vi "Red Pitaya Lockin Sweep.vi"(8 "Error In":errorcluster, 10 "Server port":u16=1002, 11 "Server address":string="192.168.1.100") -> (0 "Error Out":errorcluster)   [LabVIEW 2015]
uses:
  Mode.ctl
  Red Pitaya Parameters.ctl
  RP Command.ctl
panel:
  out "milliseconds to wait":u32=10
  in  "Desimate result":i32
  out "XY Graph":cluster{"Steps":dbl[], "Y":dbl[]}[](graph)
  out "FIFO counter":u32
  in  "Read FIFO":bool
  out "Waveform Chart 3":i32[](graph)
  out "Waveform Chart 2":i32[](graph)
  out "Waveform Chart":i32[](graph)
  out "last update, ms":i32
  in  "Controls":enum32{"Basic", "Advanced"}(tab)
  in  "Sweep":bool
  in  "Frequency step":dbl=100.0 format="%#_6p"
  in  "Stop frequency":dbl=802000.0 format="%#_6p"
  in  "Start frequency":dbl=800000.0 format="%#_6p"
  in  "Parameters":T1={"Ranges"=[20.0, 20.0], "Output frequency 1"=50000.0, "Output frequency 2"=50000.0, "Pre-trigger samples"=-100000, "Post-trigger samples"=67108864, "Desimation rate"=32, "Delayed start"=571428} {"Delayed start" format="0x%x (%d)"; "Post-trigger samples" format="0x%x (%d)"; "Pre-trigger samples" format="0x%x (%d)"; "Output frequency 2" format="%#_6p"; "Output frequency 1" format="%#_6p"; "Ranges" format="%#_12p"}
  out "CPU Temperature":dbl(slide)=48.847186279148 scale=0.0..100.0
  out "Temperature Chart":dbl(graph)=48.847186279148
  in  "Signal bits":i32=14
  in  "Read Temperature":bool=TRUE
  in  "Read trigger":bool
  in  "Start server":bool
  out "Server  output":string
  out "bytes written":i32=8
  out "Phase increment 1":u64=1717987
  out "Trigger state":bool
  in  "Mode":T2=enum."Digitizer"
  in  "Stop Server":bool
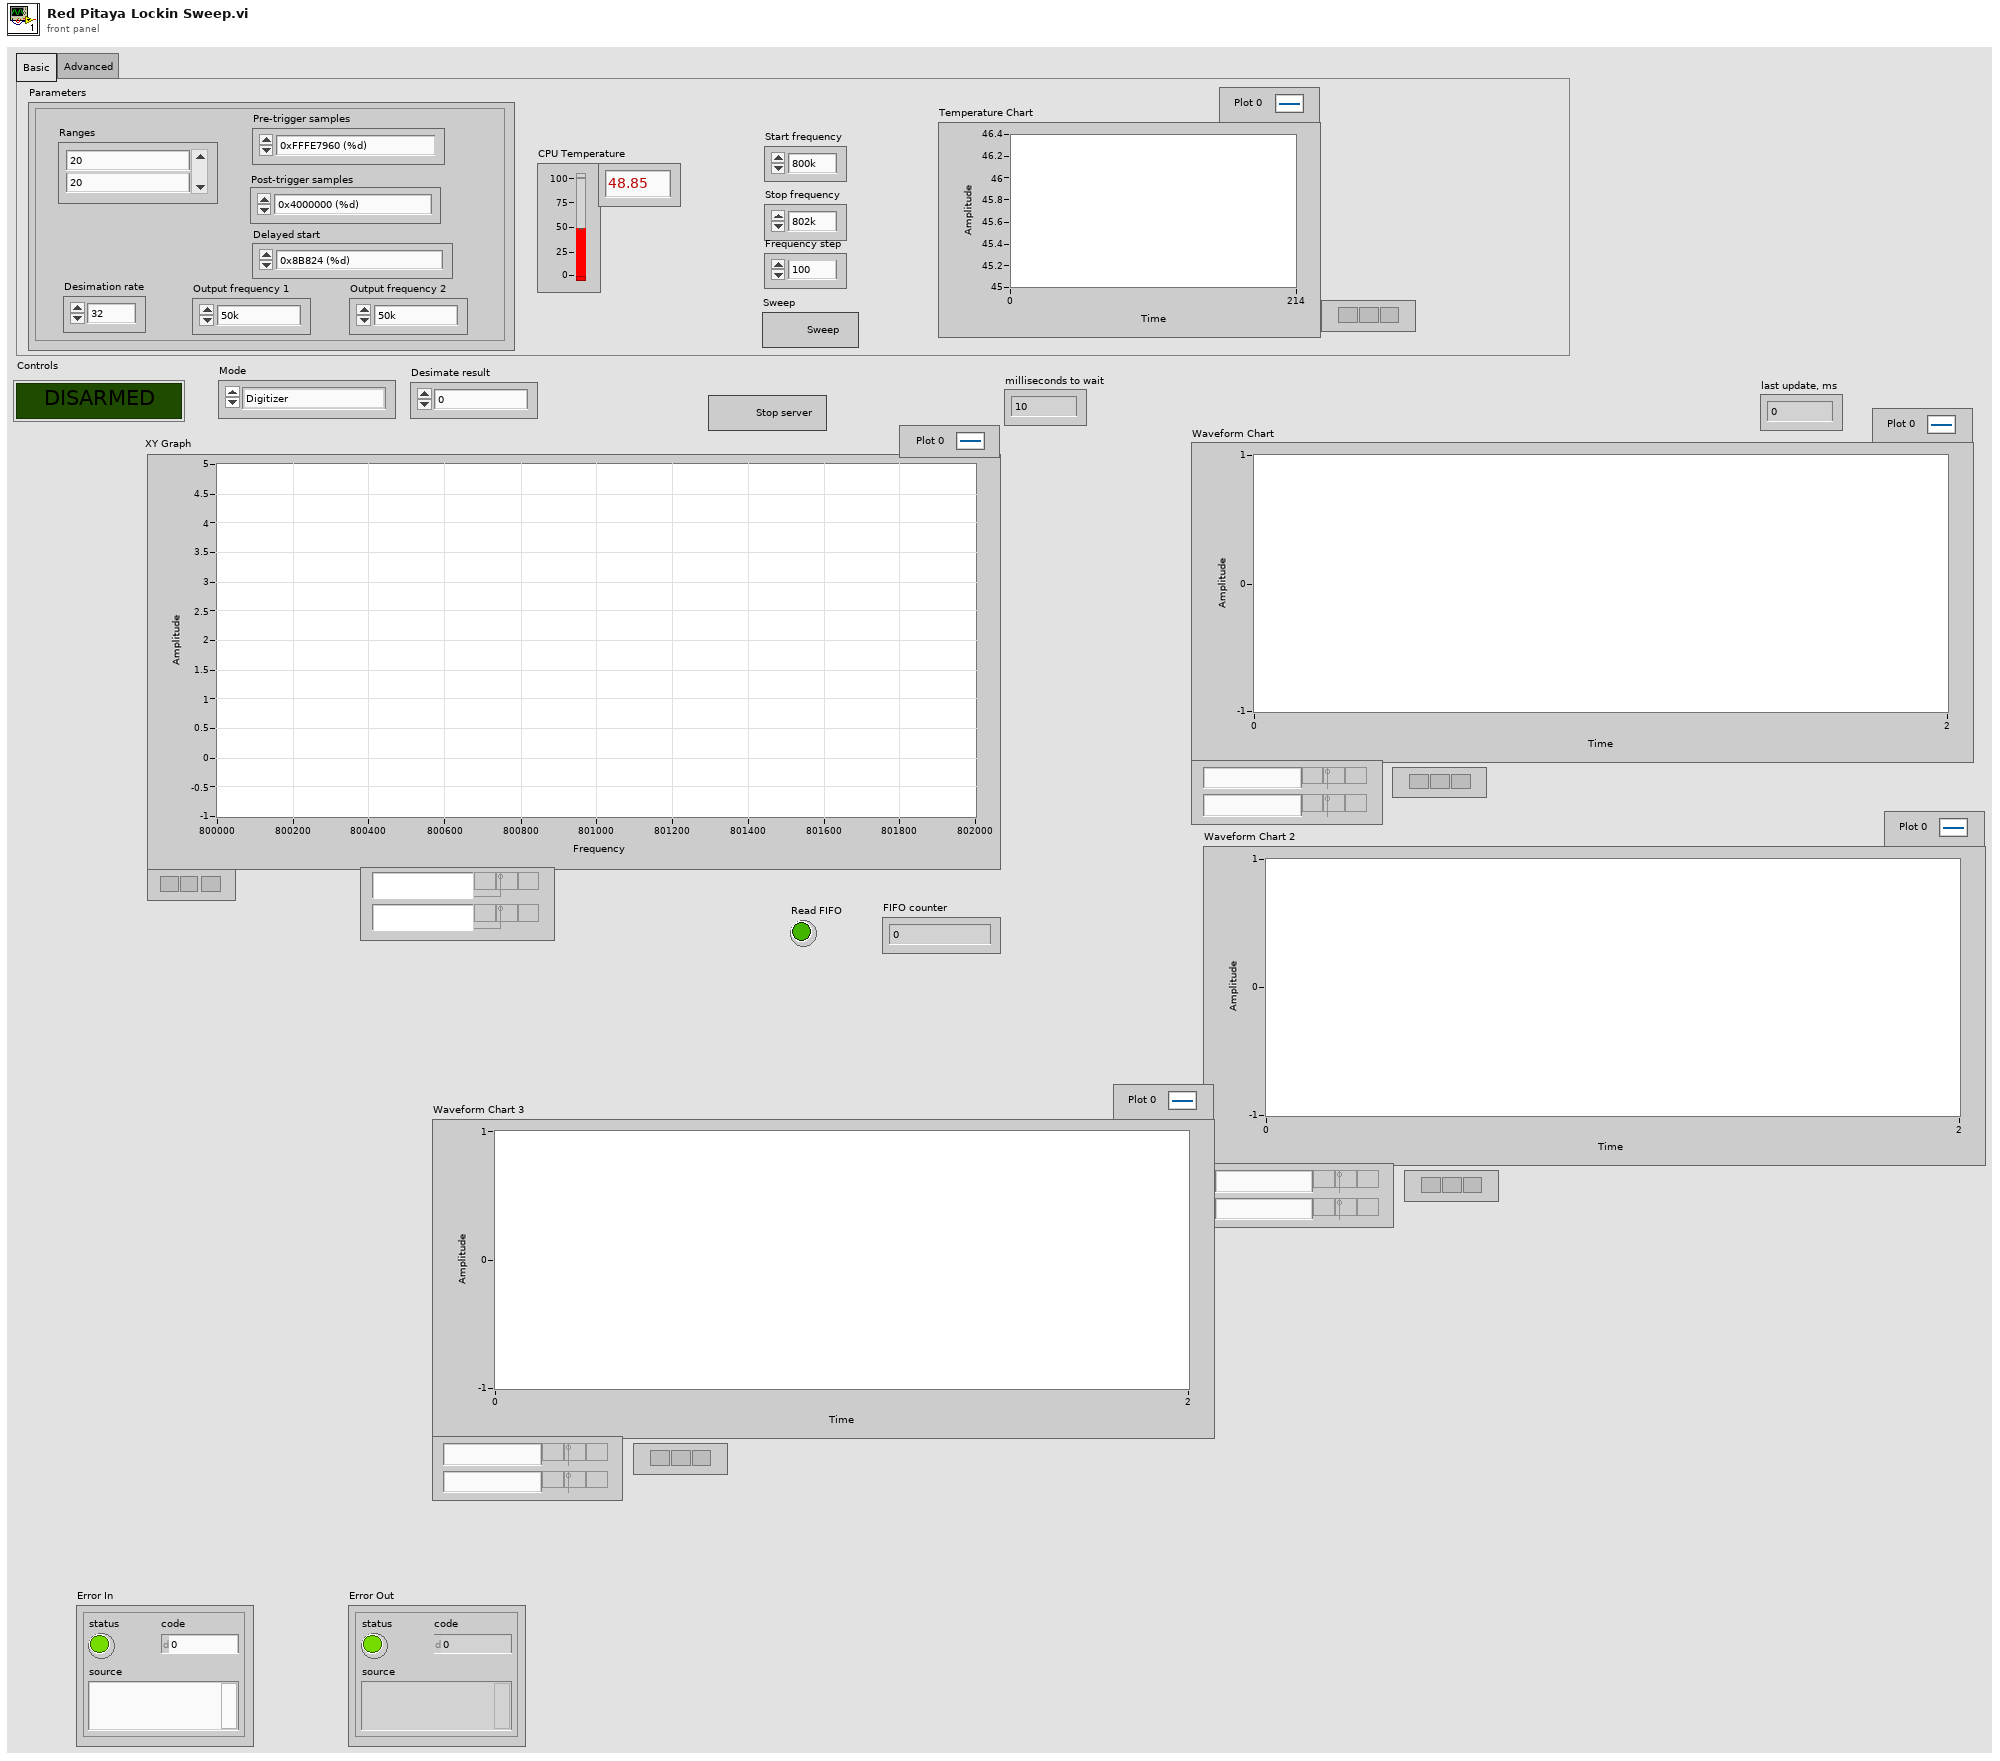
[diagram p1: front panel]
types:
  T1 = typedef "Red Pitaya Parameters.ctl" = cluster{"Ranges":dbl[], "Output frequency 1":dbl, "Output frequency 2":dbl, "Pre-trigger samples":i32, "Post-trigger samples":u64, "Desimation rate":u64, "Delayed start":u64}
  T2 = typedef "Mode.ctl" = enum16{"Filter", "Lockin test", "Snapshot test", "Digitizer", "Current-Voltage"}
  T3 = typedef "RP Command.ctl" = enum16{"Set frequency", "Arm and get data", "Stop server", "Get status", "Get temperature", "Set decimation", "Arm", "Software trigger", "Get whole buffer", "Get chunk", "System call", "Get config", "Set config", "Read FIFO", "Play pattern", "Set frequency batch"}
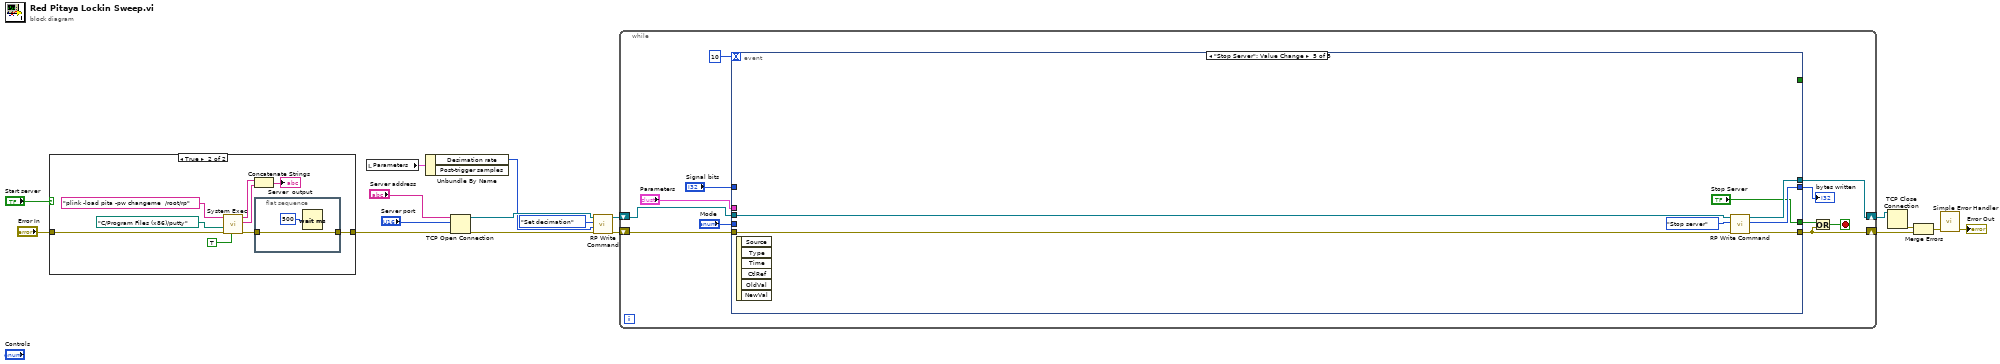
[diagram p0: block diagram]
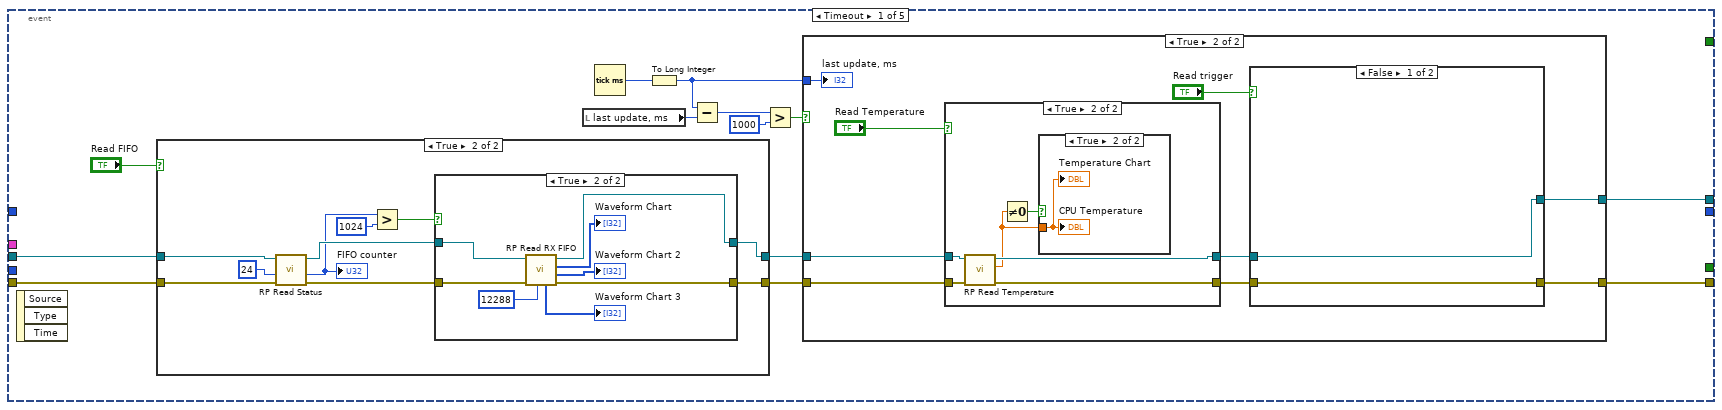
[diagram p3: hidden frame]
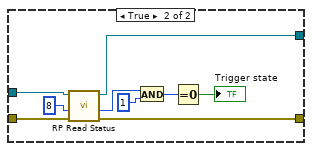
[diagram p7: hidden frame]
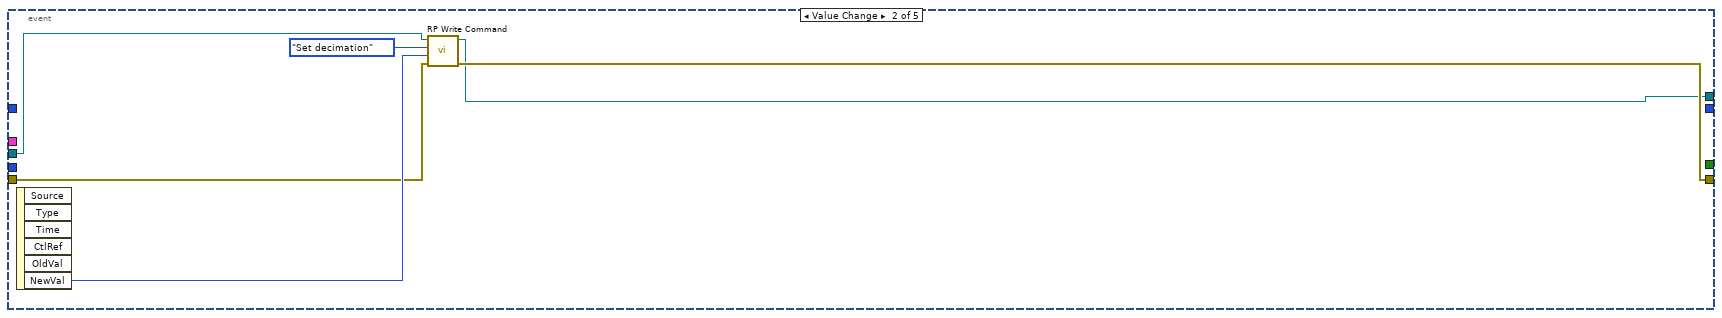
[diagram p10: hidden frame]
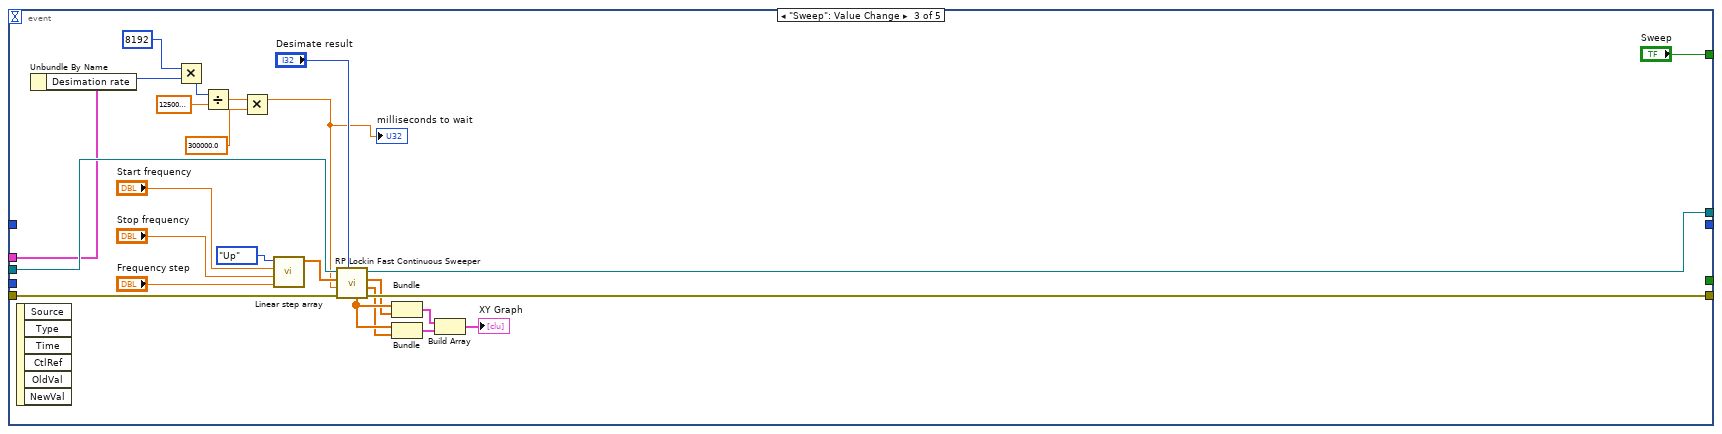
[diagram p11: hidden frame]
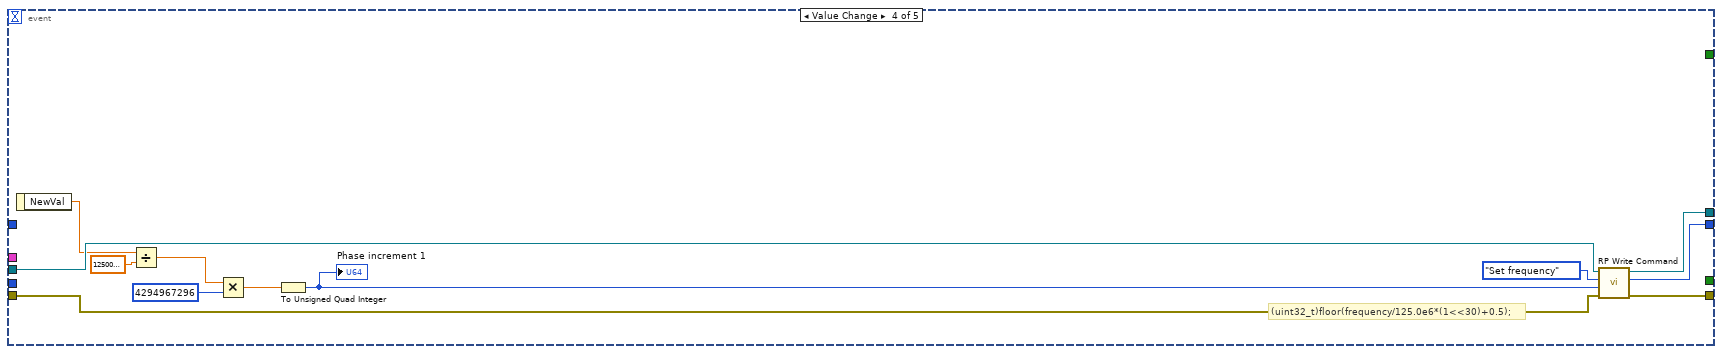
[diagram p12: hidden frame]
diagram:
  n1 = case shown="True" "Start server" {
    tunnel: [w18 w19] -> w9
    tunnel: "Error In" -> [w18 w21]
    frame False {
    }
    frame True {
      n2 = call <vilib>:"System Exec.vi"("run minimized? (F)"=TRUE, "error in (no error)"=w21, "working directory"=path "C:/Program Files (x86)/putty", "command line"="plink -load pita -pw changeme  /root/rp") -> ("error out"=w20:errorcluster, "standard error"=w23:string, "standard output"=w27:string)  [unwired: 4 in, 1 out]
      n3 = Concatenate Strings(w27, w23) -> (→"Server  output":string)
      n4 = flat-sequence {
        tunnel: w20 -> [w29]
        tunnel: [w29] -> w19
        frame #0 {
          n5 = Wait (ms)(milliseconds to wait=u32 500) -> ()  [unwired: 1 out]
        }
      }
    }
  }
  n6 = local read "Parameters"() -> (w6:T1)
  n7 = Unbundle By Name(w6) -> ("Desimation rate"=w3:u64)  [unwired: 1 out]
  n8 = TCP Open Connection(address="Server address", remote port or service name="Server port", error in (no error)=w9) -> (connection ID=w5:refnum<k5>, error out=w2:errorcluster)  [unwired: 2 in]
  n9 = call "RP Write Command.vi"("Error In"=w2, "Command payload"=w3, "Command number"=RP_Command."Set decimation", "connection ID"=w5) -> ("Error Out"=w1:errorcluster, "connection ID out"=w4:refnum<k5>)  [unwired: 5 in, 1 out]
  n10 = while {
    shift-right: [w38] -> w13
    shift-left: w4 -> [w39]
    shift-right: [w36] -> w12
    shift-left: w1 -> [w40]
    stop <- w34 stop-if-true
    n11 = event shown="[4] \"Stop Server\": Value Change" {
      selector: _ -> [_ _ _ _ _]
      dyn-events: _ -> [_ _ _ _ _]
      timeout: 10 -> [_ _ _ _ _]
      tunnel: w40 -> [w43 w110 w129 w145 w156]
      tunnel: w39 -> [w45 w109 w132 w144 w154]
      tunnel: [w53 w108 w130 w140 w153] -> w36
      tunnel: [w52 w107 w131 w141 w152] -> w38
      tunnel: [_ _ _ _ "Stop Server"] -> w35
      tunnel: [_ _ _ w139 w151] -> w37
      tunnel: "Mode" -> [_ _ _ _ _]
      tunnel: "Parameters" -> [_ _ w120 _ _]
      tunnel: "Signal bits" -> [_ _ _ _ _]
      tunnel: [_ _ "Sweep" _ _] -> _
      event Timeout {
        n12 = event-data() -> ()  [unwired: 1 in, 3 out]
        n13 = case shown="True" "Read FIFO" {
          tunnel: w45 -> [w54 w60]
          tunnel: [w54 w65] -> w44
          tunnel: w43 -> [w55 w63]
          tunnel: [w55 w64] -> w42
          frame False {
          }
          frame True {
            n14 = call "RP Read Status.vi"("Error In"=w63, "Status offset"=u64 24, "connection ID"=w60) -> ("Error Out"=w62:errorcluster, "Status response"=w58:u32, "connection ID out"=w61:refnum<k5>)  [unwired: 6 in]
            "FIFO counter" <- w58
            n15 = Greater?(x=w58, y=u32 1024) -> (0:w56:bool)
            n16 = case shown="True" w56 {
              tunnel: w61 -> [w66 w75]
              tunnel: [w66 w74] -> w65
              tunnel: [w67 w73] -> w64
              tunnel: w62 -> [w67 w69]
              frame False {
              }
              frame True {
                n17 = call "RP Read RX FIFO.vi"("FIFO Bytes per read"=12288, "Error In"=w69, "connection ID"=w75) -> ("Error Out"=w73:errorcluster, "Y"=→"Waveform Chart 2":i32[], "X"=→"Waveform Chart":i32[], "connection ID out"=w74:refnum<k5>, "F"=→"Waveform Chart 3":i32[])  [unwired: 4 in]
              }
            }
          }
        }
        n18 = local read "last update, ms"() -> (w50:i32)
        n19 = Tick Count (ms)() -> (millisecond timer value=w51:u32)
        n20 = To Long Integer(number=w51) -> (32bit integer=w46:i32)
        n21 = Subtract(x=w46, y=w50) -> (x-y=w49:i32)
        n22 = Greater?(x=w49, y=1000) -> (0:w47:bool)
        n23 = case shown="True" w47 {
          tunnel: w44 -> [w76 w85]
          tunnel: w42 -> [w77 w84]
          tunnel: [w77 w80] -> w53
          tunnel: [w76 w79] -> w52
          tunnel: w46 -> [_ w78]
          frame False {
          }
          frame True {
            n24 = case shown="True" "Read Temperature" {
              tunnel: w85 -> [w99 w104]
              tunnel: w84 -> [w98 w100]
              tunnel: [w99 w103] -> w82
              tunnel: [w98 w101] -> w81
              frame False {
              }
              frame True {
                n25 = call "RP Read Temperature.vi"("Error In"=w100, "connection ID"=w104) -> ("error out"=w101:errorcluster, "Thermometer"=w102:dbl, "connection ID out"=w103:refnum<k5>)  [unwired: 7 in]
                n26 = Not Equal To 0?(x=w102) -> (x != 0?=w105:bool)
                n27 = case shown="True" w105 {
                  tunnel: w102 -> [_ w106]
                  frame False {
                  }
                  frame True {
                    "CPU Temperature" <- w106
                    "Temperature Chart" <- w106
                  }
                }
              }
            }
            n28 = case shown="False" "Read trigger" {
              tunnel: w82 -> [w87 w96]
              tunnel: w81 -> [w88 w97]
              tunnel: [w88 w92] -> w80
              tunnel: [w87 w89] -> w79
              frame False {
              }
              frame True {
                n29 = call "RP Read Status.vi"("Error In"=w97, "Status offset"=u64 8, "connection ID"=w96) -> ("Error Out"=w92:errorcluster, "Status response"=w94:u32, "connection ID out"=w89:refnum<k5>)  [unwired: 6 in]
                n30 = And(x=w94, y=u32 1) -> (x .and. y?=w91:u32)
                n31 = Equal To 0?(x=w91) -> (x = 0?=→"Trigger state":bool)
              }
            }
            "last update, ms" <- w78
          }
        }
      }
      event Value Change {
        n32 = event-data() -> ("NewVal"=w111:u64)  [unwired: 1 in, 5 out]
        n33 = call "RP Write Command.vi"("Error In"=w110, "Command payload"=w111, "Command number"=RP_Command."Set decimation", "connection ID"=w109) -> ("Error Out"=w108:errorcluster, "connection ID out"=w107:refnum<k5>)  [unwired: 5 in, 1 out]
      }
      event "Sweep": Value Change {
        n34 = event-data() -> ()  [unwired: 1 in, 6 out]
        n35 = Unbundle By Name(w120) -> ("Desimation rate"=w119:u64)
        n36 = Multiply(x=u64 8192, y=w119) -> (x*y=w117:u64)
        n37 = Divide(x=w117, y=125000000.0) -> (x/y=w115:dbl)
        n38 = Multiply(x=w115, y=300000.0) -> (x*y=w113:dbl)
        "milliseconds to wait" <- w113
        n39 = call "Linear step array.vi"("Step"="Frequency step", "End"="Stop frequency", "Start"="Start frequency", "Mode"=enum16{"Up", "Up-down"}."Up") -> ("Steps"=w128:dbl[])  [unwired: 7 in]
        n40 = call "RP Lockin Fast Continuous Sweeper.vi"("Desimate result"="Desimate result", "Error In"=w129, "milliseconds to wait"=w113, "Frequencies"=w128, "connection ID"=w132) -> ("Error Out"=w130:errorcluster, "Y"=w122:dbl[], "X"=w123:dbl[], "connection ID out"=w131:refnum<k5>, "F"=w124:dbl[])  [unwired: 2 in]
        n41 = Bundle("F"=w124, "X"=w123) -> (w127:cluster{"F":dbl[], "X":dbl[]})  [unwired: 1 in]
        n42 = Bundle("F"=w124, "Y"=w122) -> (w126:cluster{"F":dbl[], "Y":dbl[]})  [unwired: 1 in]
        n43 = Build Array(w127, w126) -> (→"XY Graph":cluster{"F":dbl[], "Y":dbl[]}[])
      }
      event Value Change {
        # "(uint32_t)floor(frequency/125.0e6*(1<<30)+0.5);"
        n44 = event-data() -> ("NewVal"=w138:dbl)  [unwired: 1 in]
        n45 = Divide(x=w138, y=125000000.0) -> (x/y=w147:dbl)
        n46 = Multiply(x=w147, y=i64 4294967296) -> (x*y=w146:dbl)
        n47 = To Unsigned Quad Integer(1:w146) -> (0:w142:u64)
        "Phase increment 1" <- w142
        n48 = call "RP Write Command.vi"("Error In"=w145, "Command payload"=w142, "Command number"=RP_Command."Set frequency", "connection ID"=w144) -> ("Error Out"=w140:errorcluster, "bytes written"=w139:i32, "connection ID out"=w141:refnum<k5>)  [unwired: 5 in]
      }
      event "Stop Server": Value Change {
        n49 = event-data() -> ()  [unwired: 1 in, 6 out]
        n50 = call "RP Write Command.vi"("Error In"=w156, "Command number"=RP_Command."Stop server", "connection ID"=w154) -> ("Error Out"=w153:errorcluster, "bytes written"=w151:i32, "connection ID out"=w152:refnum<k5>)  [unwired: 6 in]
      }
    }
    "bytes written" <- w37
    n51 = Or(x=w35, y=w36) -> (x .or. y?=w34:bool)
  }
  n52 = TCP Close Connection(connection ID=w13) -> (error out=w15:errorcluster)  [unwired: 2 in, 1 out]
  n53 = Merge Errors(w15, w12) -> (w14:errorcluster)
  n54 = call <vilib>:"Simple Error Handler.vi"("error in (no error)"=w14) -> ("error out"=→"Error Out":errorcluster)  [unwired: 4 in, 4 out]
